vi "Set Debug Flags.vi"(10 "FIFO Debug Flags":refnum<class "FIFO Flags.lvclass">, 11 "Interface in":refnum<class "Interface.lvclass">) -> (3 "Interface out":refnum<class "Interface.lvclass">)   [LabVIEW 2017, in "DSF Core.lvlib" / "Interface.lvclass"]
uses:
  Interface.lvclass
  Debug/FIFO Flags/FIFO Flags.lvclass
  Interface.lvclass/Interface.ctl
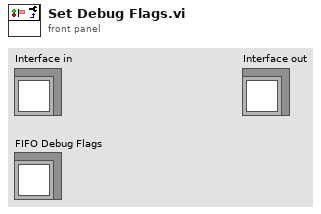
[diagram p1: front panel]
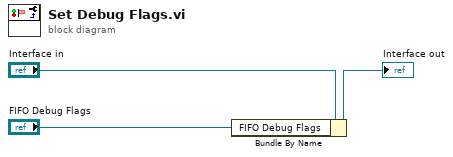
[diagram p0: block diagram]
diagram:
  n1 = Bundle By Name(cluster="Interface in", "FIFO Debug Flags"="FIFO Debug Flags") -> (→"Interface out":refnum<class "Interface.lvclass">)
